vi "Read Attributes.vi"(11 "Test Progress Msg":refnum<class "Test Progress Msg.lvclass">) -> (2 "Payload":cluster{"Test Name":string, "State":string})   [LabVIEW 2017, in "Test.lvlib" / "Test Progress Msg.lvclass"]
uses:
  Test Progress Msg.lvclass
  Test Progress Msg.lvclass/Test Progress Msg.ctl
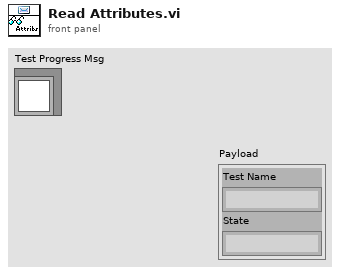
[diagram p1: front panel]
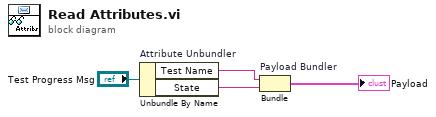
[diagram p0: block diagram]
diagram:
  n1 = Unbundle By Name "Attribute Unbundler"("Test Progress Msg") -> ("Test Name"=w2:string, "State"=w1:string)
  n2 = Bundle "Payload Bundler"("Test Name"=w2, "State"=w1) -> (→"Payload":cluster{"Test Name":string, "State":string})  [unwired: 1 in]
